vi "Configure Math Function Characteristics.vi"(0 "VISA resource name":refnum<visa-resource-name>, 1 "Vertical Offset (0.0)":dbl, 2 "Vertical Scale (10.0)":dbl=10.0, 3 "Integrate DC Offset (0.0)":dbl, 5 "Math Operation (0: Add)":i32(ring) items=["Add", "Subtract", "Multiply", "Integrate", "Diff", "FFT", "SQRT", "Magnify", "Absolute", "Square", "LN", "LOG", "EXP", "TEN", "Lowpass", "Highpass", "Divide", "Linear", "Trend", "Btiming", "Bstate", "Envelope", "Smoothing", "Max Hold", "Min Hold", "Average", "Clock Recovery"], 7 "GOFT Math Operation (0: Add)":i32(ring) items=["Add", "Subtract", "Multiply"], 9 "Enable Display (T: Enable)":bool=TRUE, 11 "error in (no error)":errorcluster, 12 "Vertical Range (8.0 V)":dbl=8.0, 13 "Vertical Scale Units (0: V)":i32(ring) items=["V", "dB"], 14 "Math Function Index (1: Math Function 1)":i32(ring)=1 items=["Math Function 1"=1, "Math Function 2"=2, "Math Function 3"=3, "Math Function 4"=4]) -> (4 "VISA resource name out":refnum<visa-resource-name>, 15 "error out":errorcluster)   [LabVIEW 2023, in "Keysight-DSQx3014T.lvlib"]
doc: "Configures the math function."
uses:
  Keysight-DSQx3014T.lvlib
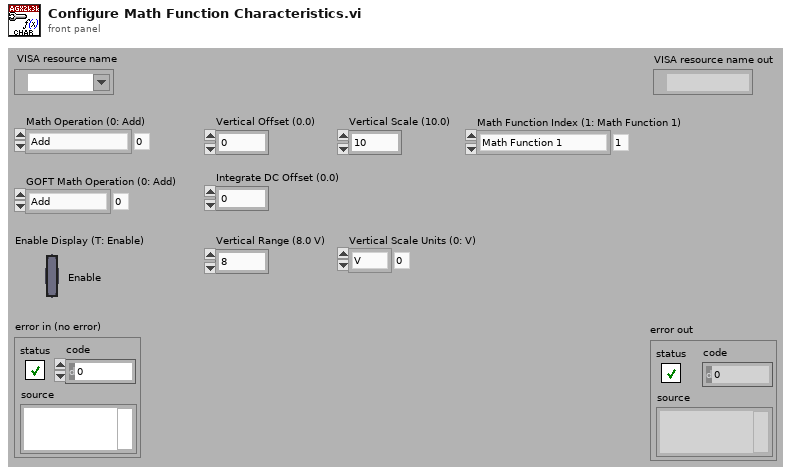
[diagram p1: front panel]
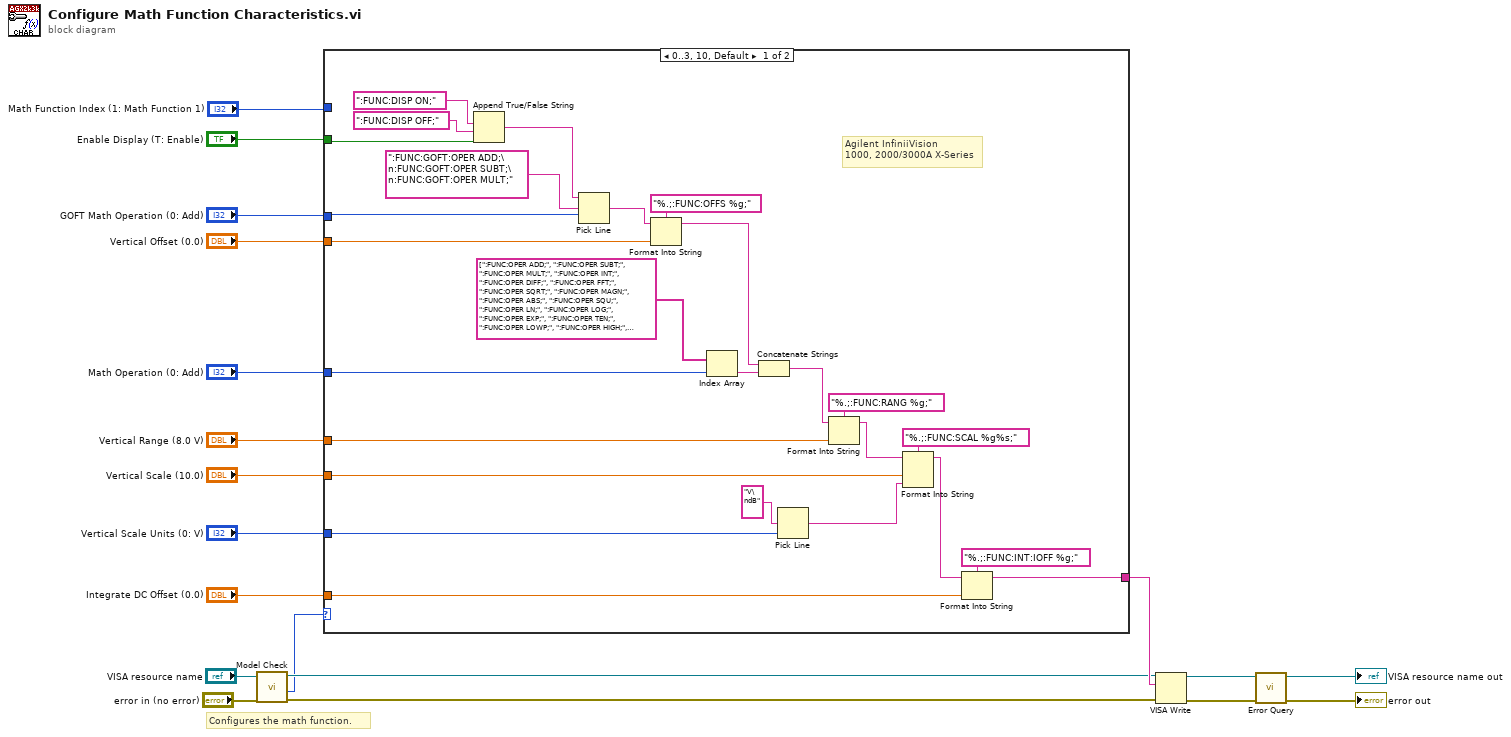
[diagram p0: block diagram]
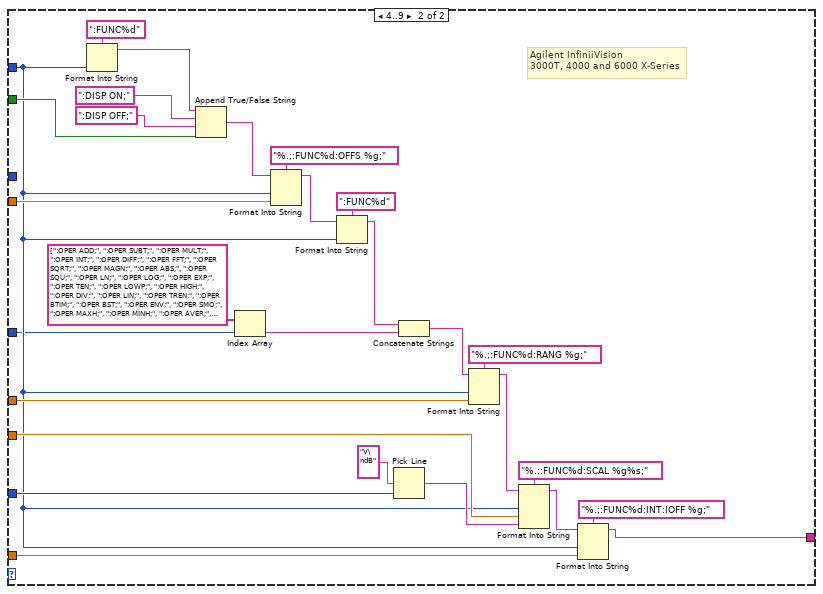
[diagram p2: hidden frame]
diagram:
  # "Configures the math function."
  n1 = call "Model Check.vi"("error in (no error)"="error in (no error)", "VISA resource name"="VISA resource name") -> ("error out"=w2:errorcluster, "Model"=w1:i32, "VISA resource name out"=w3:refnum<visa-resource-name>)  [unwired: 7 out]
  n2 = case shown="0..3, 10, Default" w1 {
    tunnel: "Enable Display (T: Enable)" -> [w28 w59]
    tunnel: "GOFT Math Operation (0: Add)" -> [w27 _]
    tunnel: "Vertical Offset (0.0)" -> [w26 w58]
    tunnel: "Math Operation (0: Add)" -> [w25 w48]
    tunnel: "Vertical Range (8.0 V)" -> [w24 w57]
    tunnel: "Vertical Scale (10.0)" -> [w23 w54]
    tunnel: "Vertical Scale Units (0: V)" -> [w22 w55]
    tunnel: "Integrate DC Offset (0.0)" -> [w21 w53]
    tunnel: "Math Function Index (1: Math Function 1)" -> [_ w50]
    tunnel: [w20 w47] -> w6
    frame 0..3, 10, Default {
      # "Agilent InfiniiVision\n1000, 2000/3000A X-Series"
      n3 = Append True/False String(1:w28, 2:":FUNC:DISP OFF;", 3:":FUNC:DISP ON;") -> (0:w42:string)  [unwired: 1 out]
      n4 = Pick Line(string ("")=w42, multi-line string=":FUNC:GOFT:OPER ADD;\n:FUNC:GOFT:OPER SUBT;\n:FUNC:GOFT:OPER MULT;", line index=w27) -> (output string=w41:string)
      n5 = Format Into String(format string="%.;:FUNC:OFFS %g;", initial string=w41, w26) -> (resulting string=w32:string)  [unwired: 1 in, 1 out]
      n6 = Index Array(array=string[] [":FUNC:OPER ADD;", ":FUNC:OPER SUBT;", ":FUNC:OPER MULT;", ":FUNC:OPER INT;", ":FUNC:OPER DIFF;", ":FUNC:OPER FFT;", ":FUNC:OPER SQRT;", ":FUNC:OPER MAGN;", ":FUNC:OPER ABS;", ":FUNC:OPER SQU;", ":FUNC:OPER LN;", ":FUNC:OPER LOG;", ":FUNC:OPER EXP;", ":FUNC:OPER TEN;", ":FUNC:OPER LOWP;", ":FUNC:OPER HIGH;", ":FUNC:OPER DIV;", ":FUNC:OPER LIN;", ":FUNC:OPER TREN;", ":FUNC:OPER BTIM;", ":FUNC:OPER BST;", ":FUNC:OPER ENV;\n", ":FUNC:OPER SMO;", ":FUNC:OPER MAXH;", ":FUNC:OPER MINH;", ""], index=w25) -> (element=w33:string)
      n7 = Concatenate Strings(w32, w33) -> (w31:string)
      n8 = Pick Line(multi-line string="V\ndB", line index=w22) -> (output string=w35:string)  [unwired: 1 out]
      n9 = Format Into String(format string="%.;:FUNC:RANG %g;", initial string=w31, w24) -> (resulting string=w37:string)  [unwired: 1 in, 1 out]
      n10 = Format Into String(format string="%.;:FUNC:SCAL %g%s;", initial string=w37, w23, w35) -> (resulting string=w29:string)  [unwired: 1 in, 1 out]
      n11 = Format Into String(format string="%.;:FUNC:INT:IOFF %g;", initial string=w29, w21) -> (resulting string=w20:string)  [unwired: 1 in, 1 out]
    }
    frame 4..9 {
      # "Agilent InfiniiVision\n3000T, 4000 and 6000 X-Series"
      n12 = Format Into String(format string=":FUNC%d", w50) -> (resulting string=w60:string)  [unwired: 2 in, 1 out]
      n13 = Append True/False String(1:w59, 2:":DISP OFF;", 3:":DISP ON;", 4:w60) -> (0:w46:string)
      n14 = Index Array(array=string[] [":OPER ADD;", ":OPER SUBT;", ":OPER MULT;", ":OPER INT;", ":OPER DIFF;", ":OPER FFT;", ":OPER SQRT;", ":OPER MAGN;", ":OPER ABS;", ":OPER SQU;", ":OPER LN;", ":OPER LOG;", ":OPER EXP;", ":OPER TEN;", ":OPER LOWP;", ":OPER HIGH;", ":OPER DIV;", ":OPER LIN;", ":OPER TREN;", ":OPER BTIM;", ":OPER BST;", ":OPER ENV;", ":OPER SMO;", ":OPER MAXH;", ":OPER MINH;", ":OPER AVER;", ":OPER CLOCK;"], index=w48) -> (element=w65:string)
      n15 = Format Into String(format string="%.;:FUNC%d:OFFS %g;", initial string=w46, w50, w58) -> (resulting string=w51:string)  [unwired: 1 in, 1 out]
      n16 = Format Into String(format string=":FUNC%d", initial string=w51, w50) -> (resulting string=w49:string)  [unwired: 1 in, 1 out]
      n17 = Pick Line(multi-line string="V\ndB", line index=w55) -> (output string=w56:string)  [unwired: 1 out]
      n18 = Concatenate Strings(w49, w65) -> (w64:string)
      n19 = Format Into String(format string="%.;:FUNC%d:RANG %g;", initial string=w64, w50, w57) -> (resulting string=w68:string)  [unwired: 1 in, 1 out]
      n20 = Format Into String(format string="%.;:FUNC%d:SCAL %g%s;", initial string=w68, w50, w54, w56) -> (resulting string=w62:string)  [unwired: 1 in, 1 out]
      n21 = Format Into String(format string="%.;:FUNC%d:INT:IOFF %g;", initial string=w62, w50, w53) -> (resulting string=w47:string)  [unwired: 1 in, 1 out]
    }
  }
  n22 = VISA Write(VISA resource name=w3, write buffer=w6, error in (no error)=w2) -> (VISA resource name out=w19:refnum<visa-resource-name>, error out=w18:errorcluster)  [unwired: 1 out]
  n23 = call "Error Query.vi"("error in (no error)"=w18, "VISA resource name"=w19) -> ("error out"=→"error out":errorcluster, "VISA resource name out"=→"VISA resource name out":refnum<visa-resource-name>)  [unwired: 8 out]
